vi "Complex_FFT.vi"() -> ()   [LabVIEW 2009]
uses:
  <vilib>/imath/engines/lvmath2/RunTimeEngine/ErrorHandling/NIMS_Finalize Error.vi
  <vilib>/imath/engines/lvmath2/RunTimeEngine/Parser/MC_Version.vi
  <vilib>/imath/engines/lvmath2/RunTimeEngine/NodeEndStatement/NIMS_NodeEndStatement_Output.vi
  <instcachedir>/0/NIMS_NodeEndStatement_Output_53EC0D466D134D7ABD903AC30B43404B.lvgen/NIMS_NodeEndStatement_Output_53EC0D466D134D7ABD903AC30B43404B_001.vi
  <vilib>/imath/engines/lvmath2/RunTimeEngine/RangeToken/NIMS_Range.vi
  <instcachedir>/0/NIMS_Range_08574DECC23E450FAF0AC0BC39E6BEA7.lvgen/NIMS_Range_08574DECC23E450FAF0AC0BC39E6BEA7_000.vi
  <vilib>/imathl/engines/lvmath/Functions/Error Handling/Create Error.vi
  <vilib>/imath/engines/lvmath2/RunTimeEngine/ArithmeticOperatorToken/NIMS_ArithmeticOperator_times.vi
  <instcachedir>/0/NIMS_ArithmeticOperator_times_7E710EE12B7B45F08AF5427E7FF1D6D8.lvgen/NIMS_ArithmeticOperator_times_7E710EE12B7B45F08AF5427E7FF1D6D8_001.vi
  <vilib>/imath/engines/lvmath2/RunTimeEngine/ArithmeticOperatorToken/NIMS_ArithmeticOperator_plus.vi
  <instcachedir>/0/NIMS_ArithmeticOperator_plus_48B9519178ED42D7840F01273E784BFE.lvgen/NIMS_ArithmeticOperator_plus_48B9519178ED42D7840F01273E784BFE_002.vi
  <vilib>/imath/engines/lvmath/Functions/Error Handling/MergeErrorsWrapper.vi
  <vilib>/imath/engines/lvmath/Functions/Error Handling/MC_Error Cluster From Error Code.vi
  <vilib>/imath/engines/lvmath2/RunTimeEngine/BuiltInFunctions/randnormal/NIMS_randnormal(1,I32).vi
  <vilib>/imath/engines/lvmath2/RunTimeEngine/ArithmeticOperatorToken/NIMS_ArithmeticOperator_power(S).vi
  <instcachedir>/0/NIMS_ArithmeticOperator_power(S)_4AA2794EBDEE41D3AEDF40937D3906E7.lvgen/NIMS_ArithmeticOperator_power(S)_4AA2794EBDEE41D3AEDF40937D3906E7_001.vi
  <instcachedir>/0/NIMS_ArithmeticOperator_plus_48B9519178ED42D7840F01273E784BFE.lvgen/NIMS_ArithmeticOperator_plus_48B9519178ED42D7840F01273E784BFE_003.vi
  <vilib>/imath/engines/lvmath2/RunTimeEngine/BuiltInFunctions/clfig/NIMS_clfig.vi
  <vilib>/imath/engines/lvmath2/RunTimeEngine/BuiltInFunctions/fft/NIMS_fft(GV).vi
  <instcachedir>/0/NIMS_fft(GV)_4C6467FC22F84E4BA42517A07EF978B0.lvgen/NIMS_fft(GV)_4C6467FC22F84E4BA42517A07EF978B0_000.vi
  <vilib>/imath/engines/lvmath2/RunTimeEngine/BuiltInFunctions/abs/NIMS_abs(signed).vi
  <instcachedir>/0/NIMS_abs(signed)_C4FCB8E6058B49B797C7C8D53CA5F6EC.lvgen/NIMS_abs(signed)_C4FCB8E6058B49B797C7C8D53CA5F6EC_000.vi
  <vilib>/imath/engines/lvmath2/RunTimeEngine/BuiltInFunctions/max/1 input/NIMS_max(CV).vi
  <instcachedir>/0/NIMS_max(CV)_9563C82345104A5B930680B94D5C7A1A.lvgen/NIMS_max(CV)_9563C82345104A5B930680B94D5C7A1A_000.vi
  <vilib>/imath/engines/lvmath2/RunTimeEngine/BuiltInFunctions/length/NIMS_length(GV).vi
  <instcachedir>/0/NIMS_length(GV)_08A3D13377FD4E4B96F5795FBF3698FA.lvgen/NIMS_length(GV)_08A3D13377FD4E4B96F5795FBF3698FA_001.vi
panel:
  out "XY Graph 2":cluster{dbl[], dbl[]}(graph)
  out "XY Graph":cluster{dbl[], dbl[]}(graph)
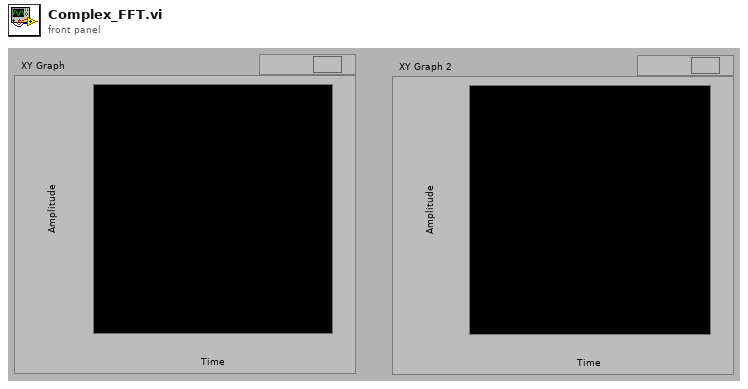
[diagram p1: front panel]
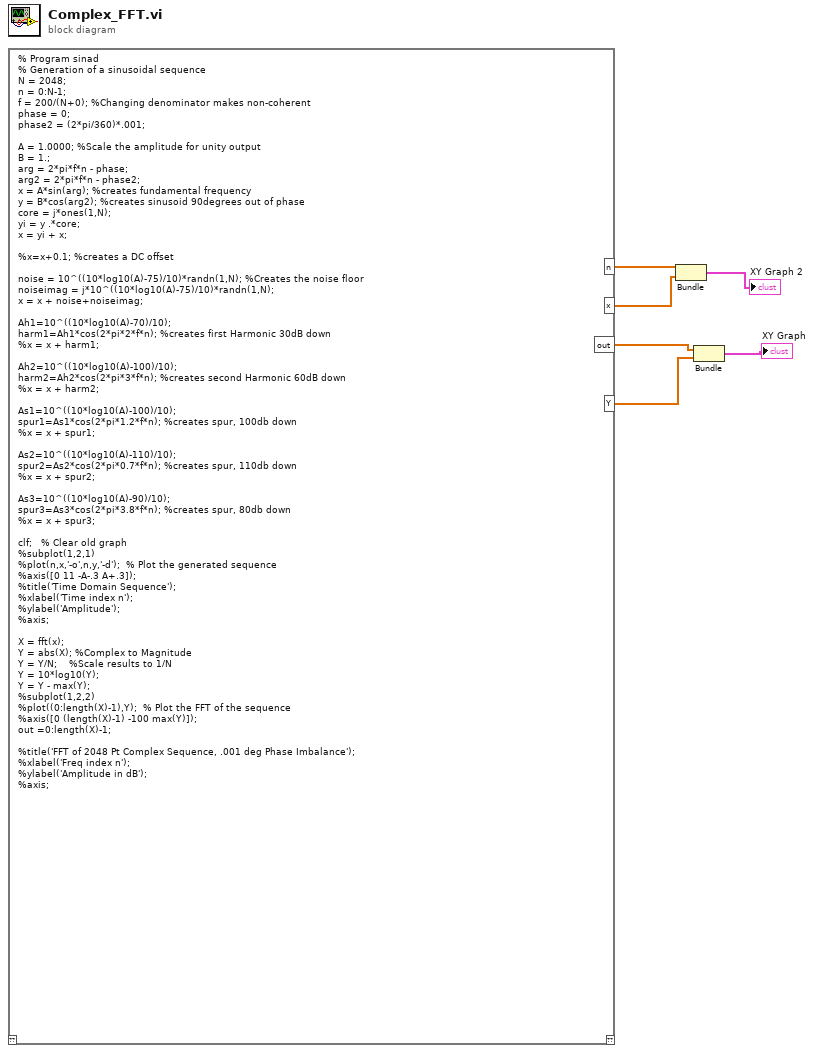
[diagram p0: block diagram]
diagram:
  n1 = mathscript code="% Program sinad\n% Generation of a sinusoidal sequence\nN = 2048;\nn = 0:N-1;\t\nf = 200/(N+0); %Changing denominator makes non-coherent\nphase = 0;\t\nphase2 = (2*pi/360)*.001;\n\nA = 1.0000; %Scale the amplitude for unity output\nB = 1.;\narg = 2*pi*f*n - phase; \narg2 = 2*pi*f*n - phase2;\nx = A*sin(arg); %creates fundamental frequency\ny = B*cos(arg2); %creates sinusoid 90degrees out of phase\ncore = j*ones(1,N);\nyi = y .*core;\nx = yi + x;\n\n%x=x+0.1; %creates a DC offset\n\nnoise = 10^((10*log10(A)-75)/10)*randn(1,N); %Creates the noise floor\nnoiseimag = j*10^((10*log10(A)-75)/10)*randn(1,N);\nx = x + noise+noiseimag;\n\nAh1=10^((10*log10(A)-70)/10);\nharm1=Ah1*cos(2*pi*2*f*n); %creates first Harmonic 30dB down\n%x = x + harm1;\n\nAh2=10^((10*log10(A)-100)/10);\nharm2=Ah2*cos(2*pi*3*f*n); %creates second Harmonic 60dB down\n%x = x + harm2;\n\nAs1=10^((10*log10(A)-100)/10);\nspur1=As1*cos(2*pi*1.2*f*n); %creates spur, 100db down\n%x = x + spur1;\n\nAs2=10^((10*log10(A)-110)/10);\nspur2=As2*cos(2*pi*0.7*f*n); %creates spur, 110db down\n%x = x + spur2;\n\nAs3=10^((10*log10(A)-90)/10);\nspur3=As3*cos(2*pi*3.8*f*n); %creates spur, 80db down\n%x = x + spur3;\n\nclf;\t\t\t% Clear old graph\n%subplot(1,2,1)\n%plot(n,x,'-o',n,y,'-d');\t\t% Plot the generated sequence\n%axis([0 11 -A-.3 A+.3]);\n%title('Time Domain Sequence');\n%xlabel('Time index n');\n%ylabel('Amplitude');\n%axis;\n\nX = fft(x);\nY = abs(X); %Complex to Magnitude\nY = Y/N;    %Scale results to 1/N\nY = 10*log10(Y);\nY = Y - max(Y);\n%subplot(1,2,2)\n%plot((0:length(X)-1),Y);\t\t% Plot the FFT of the sequence\n%axis([0 (length(X)-1) -100 max(Y)]);\nout =0:length(X)-1;\n \n%title('FFT of 2048 Pt Complex Sequence, .001 deg Phase Imbalance');\n%xlabel('Freq index n');\n%ylabel('Amplitude in dB');\n%axis;"() -> ("n"=w6:dbl[], "x"=w5:dbl[], "Y"=w2:dbl[], "out"=w3:dbl[])  [unwired: 1 in, 1 out]
  n2 = Bundle(w6, w5) -> (→"XY Graph 2":cluster{dbl[], dbl[]})  [unwired: 1 in]
  n3 = Bundle(w3, w2) -> (→"XY Graph":cluster{dbl[], dbl[]})  [unwired: 1 in]
